vi "getPath.vi"(8 "error in (no error)":errorcluster, 11 "Waypoint in":refnum<class "Waypoint.lvclass">) -> (0 "error out":errorcluster, 2 "Path":T1[](array[typedef]), 3 "Waypoint out":refnum<class "Waypoint.lvclass">)   [LabVIEW 2014, in "Waypoint.lvclass"]
uses:
  <userlib>/AdvancedDataStructures/ClassBased/Applications/RouteSearch/Waypoint/Waypoint.lvclass
  <userlib>/AdvancedDataStructures/ClassBased/Applications/RouteSearch/Waypoint/point.ctl
  <userlib>/AdvancedDataStructures/ClassBased/Applications/RouteSearch/Waypoint/Waypoint.lvclass/Waypoint.ctl
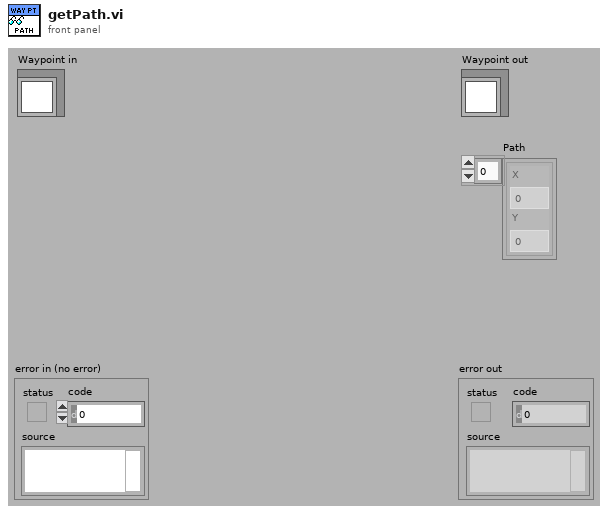
[diagram p1: front panel]
types:
  T1 = typedef "Waypoint.lvclass/point.ctl" = cluster{"X":dbl, "Y":dbl}
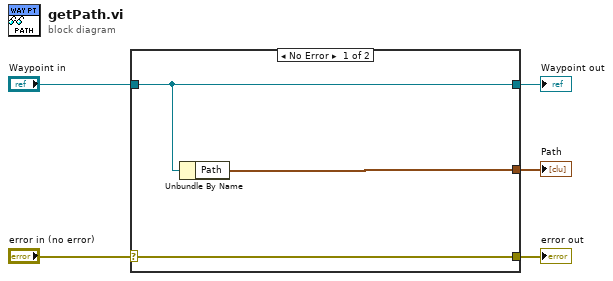
[diagram p0: block diagram]
diagram:
  n1 = case shown="No Error" "error in (no error)" {
    selector: "error in (no error)" -> [w8 w9]
    tunnel: [w8 w9] -> w4
    tunnel: [w7 w10] -> w2
    tunnel: "Waypoint in" -> [w7 w10]
    tunnel: [w6 _] -> w1
    frame No Error {
      n2 = Unbundle By Name(w7) -> ("Path"=w6:T1[])
    }
    frame Error {
    }
  }
  "error out" <- w4
  "Waypoint out" <- w2
  "Path" <- w1
